vi "PCert-Container-StoreGlbDBAdrs.vi"(8 "error in (no error)":errorcluster, 10 "DB Address":string, 11 "ERP-Container-UI in":refnum<class "PCert-Container-UI.lvclass">) -> (0 "error out":errorcluster, 3 "ERP-Container-UI out":refnum<class "PCert-Container-UI.lvclass">)   [LabVIEW 2013, in "PCert-Container-UI.lvclass"]
uses:
  PCert-Container-UI.lvclass
  PCert-Container-UI.lvclass/PCert-Container-UI.ctl
  ftw-dataflow/Core/src/Database/FTW-SQLite-Connector.lvclass
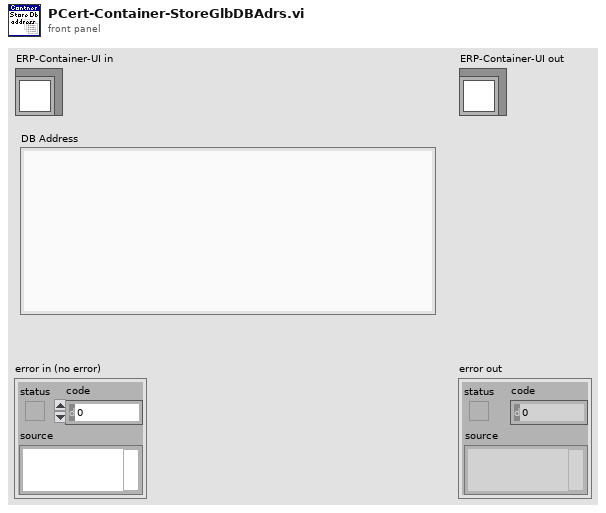
[diagram p1: front panel]
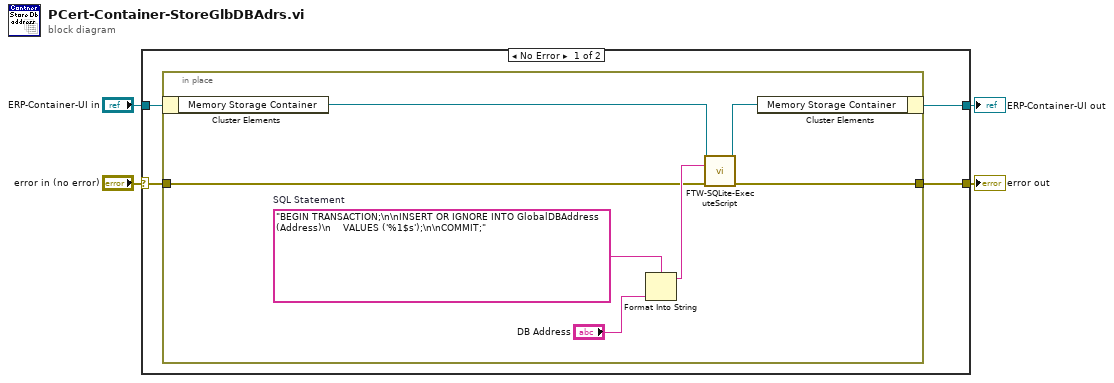
[diagram p0: block diagram]
diagram:
  n1 = case shown="No Error" "error in (no error)" {
    selector: "error in (no error)" -> [w8 w17]
    tunnel: [w7 w17] -> w3
    tunnel: [w5 w16] -> w1
    tunnel: "ERP-Container-UI in" -> [w6 w16]
    frame No Error {
      n2 = in-place {
        in-place-border: w8 -> [w10]
        in-place-border: [w9] -> w7
        w14 = "BEGIN TRANSACTION;\n\nINSERT OR IGNORE INTO GlobalDBAddress (Address)\n    VALUES ('%1$s');\n\nCOMMIT;"  # SQL Statement
        n3 = in-place-cluster #1(w6) -> ("Memory Storage Container"=w11:refnum<class "FTW-SQLite-Connector.lvclass">)
        n4 = Format Into String(format string=w14, "DB Address") -> (resulting string=w13:string)  [unwired: 2 in, 1 out]
        n5 = call "FTW-SQLite-ExecuteScript.vi"("SQLite Connector"=w11, "SQL Script"=w13, "error in"=w10) -> ("SQLite Connector out"=w12:refnum<class "FTW-SQLite-Connector.lvclass">, "error out"=w9:errorcluster)  [unwired: 9 in, 2 out]
        n6 = in-place-cluster #1("Memory Storage Container"=w12) -> (w5:refnum<class "PCert-Container-UI.lvclass">)
      }
    }
    frame Error {
    }
  }
  "error out" <- w3
  "ERP-Container-UI out" <- w1
